vi "Julian_project2.vi"() -> ()   [LabVIEW 2020]
uses:
  Control 2.ctl
panel:
  out "Numeric 2":dbl
  out "Numeric":dbl
  out "Total":i32
  out "Time":dbl
  in  "Cluster":T1
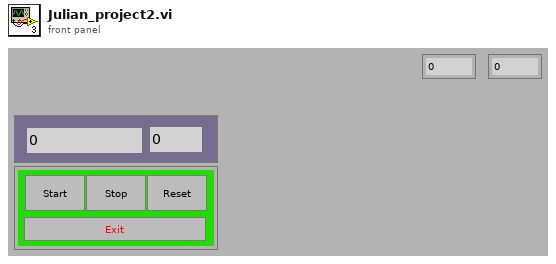
[diagram p1: front panel]
types:
  T1 = cluster{"Stop":bool, "Reset":bool, "Exit":bool, "Start":bool}
  T2 = typedef "Control 2.ctl" = enum16{"idle", "Run", "wait", "reset"}
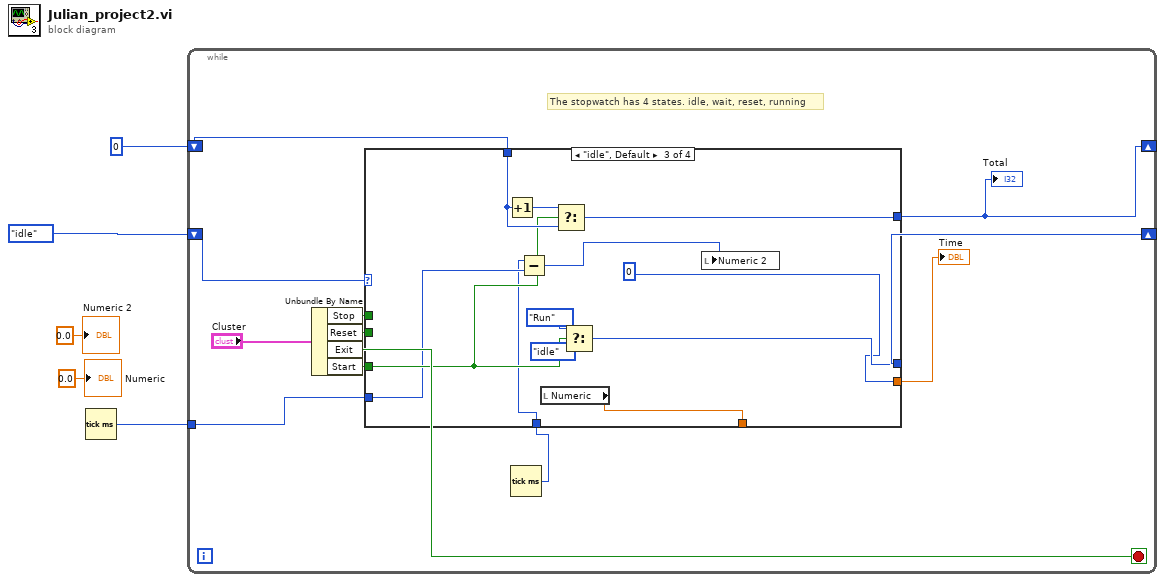
[diagram p0: block diagram]
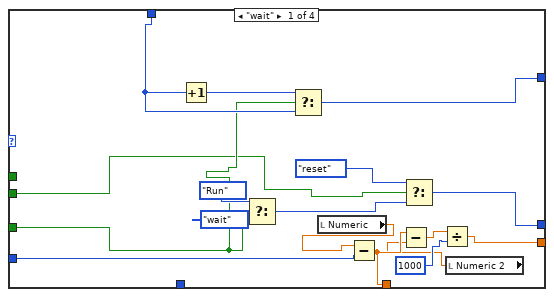
[diagram p2: hidden frame]
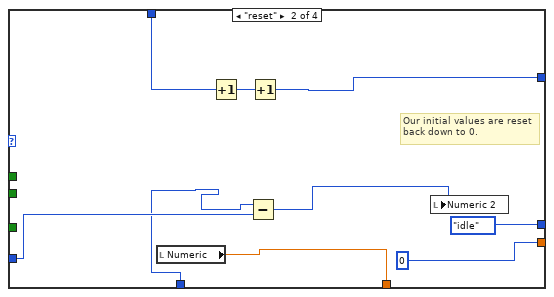
[diagram p3: hidden frame]
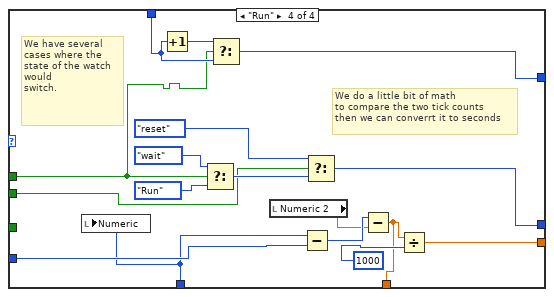
[diagram p4: hidden frame]
diagram:
  n1 = Tick Count (ms)() -> (millisecond timer value=w3:u32)
  n2 = while {
    tunnel: w3 -> [w6]
    shift-right: [w11] -> _
    shift-left: Control_2."idle" -> [w15]
    shift-right: [w9] -> _
    shift-left: 0 -> [w10]
    stop <- w16 stop-if-true
    # "The stopwatch has 4 states. idle, wait, reset, running"
    n3 = Unbundle By Name("Cluster") -> ("Stop"=w14:bool, "Reset"=w13:bool, "Exit"=w16:bool, "Start"=w12:bool)
    n4 = Tick Count (ms)() -> (millisecond timer value=w7:u32)
    n5 = case shown="\"idle\", Default" w15 {
      tunnel: w14 -> [_ _ _ w63]
      tunnel: w13 -> [w27 _ _ w64]
      tunnel: [w25 Control_2."idle" w53 w68] -> w11
      tunnel: w12 -> [w30 _ w49 _]
      tunnel: w10 -> [w31 w42 w51 w66]
      tunnel: [w33 w40 w50 w65] -> w9
      tunnel: w6 -> [w24 w38 w45 w62]
      tunnel: [w21 0 u32 0 ("x") w60] -> w8
      tunnel: w7 -> [_ w37 w44 w56]
      tunnel: [w20 w39 w48 w57] -> _
      frame "wait" {
        n6 = Increment(x=w31) -> (x+1=w32:i32)
        n7 = Select(t=Control_2."Run", s=w30, f=Control_2."wait") -> (s? t:f=w26:T2)
        n8 = Select(t=w32, s=w30, f=w31) -> (s? t:f=w33:i32)
        n9 = local read "Numeric"() -> (w23:dbl)
        n10 = Subtract(x=w23, y=w24) -> (x-y=w20:dbl)
        n11 = Select(t=Control_2."reset", s=w27, f=w26) -> (s? t:f=w25:T2)
        n12 = local read "Numeric 2"() -> (w18:dbl)
        n13 = Subtract(x=w20, y=w18) -> (x-y=w19:dbl)
        n14 = Divide(x=w19, y=1000) -> (x/y=w21:dbl)
      }
      frame "reset" {
        # "Our initial values are reset\nback down to 0."
        n15 = local read "Numeric"() -> (w39:dbl)
        n16 = Increment(x=w42) -> (x+1=w41:i32)
        n17 = Subtract(x=w37, y=w38) -> (x-y=w36:u32)
        n18 = Increment(x=w41) -> (x+1=w40:i32)
        n19 = local write "Numeric 2"(w36) -> ()
      }
      frame "idle", Default {
        n20 = Increment(x=w51) -> (x+1=w52:i32)
        n21 = Subtract(x=w44, y=w45) -> (x-y=w46:u32)
        n22 = local read "Numeric"() -> (w48:dbl)
        n23 = Select(t=w52, s=w49, f=w51) -> (s? t:f=w50:i32)
        n24 = Select(t=Control_2."Run", s=w49, f=Control_2."idle") -> (s? t:f=w53:T2)
        n25 = local write "Numeric 2"(w46) -> ()
      }
      frame "Run" {
        # "We have several\ncases where the \nstate of the watch would \nswitch."
        # "We do a little bit of math \nto compare the two tick counts\nthen we can converrt it to seconds"
        n26 = local write "Numeric"(w56) -> ()
        n27 = Increment(x=w66) -> (x+1=w67:i32)
        n28 = Select(t=Control_2."wait", s=w63, f=Control_2."Run") -> (s? t:f=w70:T2)
        n29 = Select(t=w67, s=w63, f=w66) -> (s? t:f=w65:i32)
        n30 = local read "Numeric 2"() -> (w58:dbl)
        n31 = Subtract(x=w56, y=w62) -> (x-y=w59:u32)
        n32 = Select(t=Control_2."reset", s=w64, f=w70) -> (s? t:f=w68:T2)
        n33 = Subtract(x=w59, y=w58) -> (x-y=w57:dbl)
        n34 = Divide(x=w57, y=1000) -> (x/y=w60:dbl)
      }
    }
    "Time" <- w8
    "Total" <- w9
  }
  "Numeric 2" <- 0.0 ("Numeric 2")
  "Numeric" <- 0.0 ("Numeric")
